vi "PvgeneratorOP400.vi"(8 "errin":errorcluster, 9 "BDD 3":T1, 10 "network":path, 11 "path in":path) -> (0 "sortie d'erreur":errorcluster caption="errout", 1 "network out":path, 2 "tout bon":bool, 3 "Chaîne":string)   [LabVIEW 2020]
uses:
  VG/IS30%.vi
  VG/PN.vi
  SubVI/OP400ZP_OCVmin.vi
  SubVI/OP400ZP_OCVmax.vi
  <vilib>/Utility/config.llb/NI_LVConfig.lvlib
panel:
  out "BDD 2":T2
  out "BDD":T1
  out "nombre de remplacements":i32
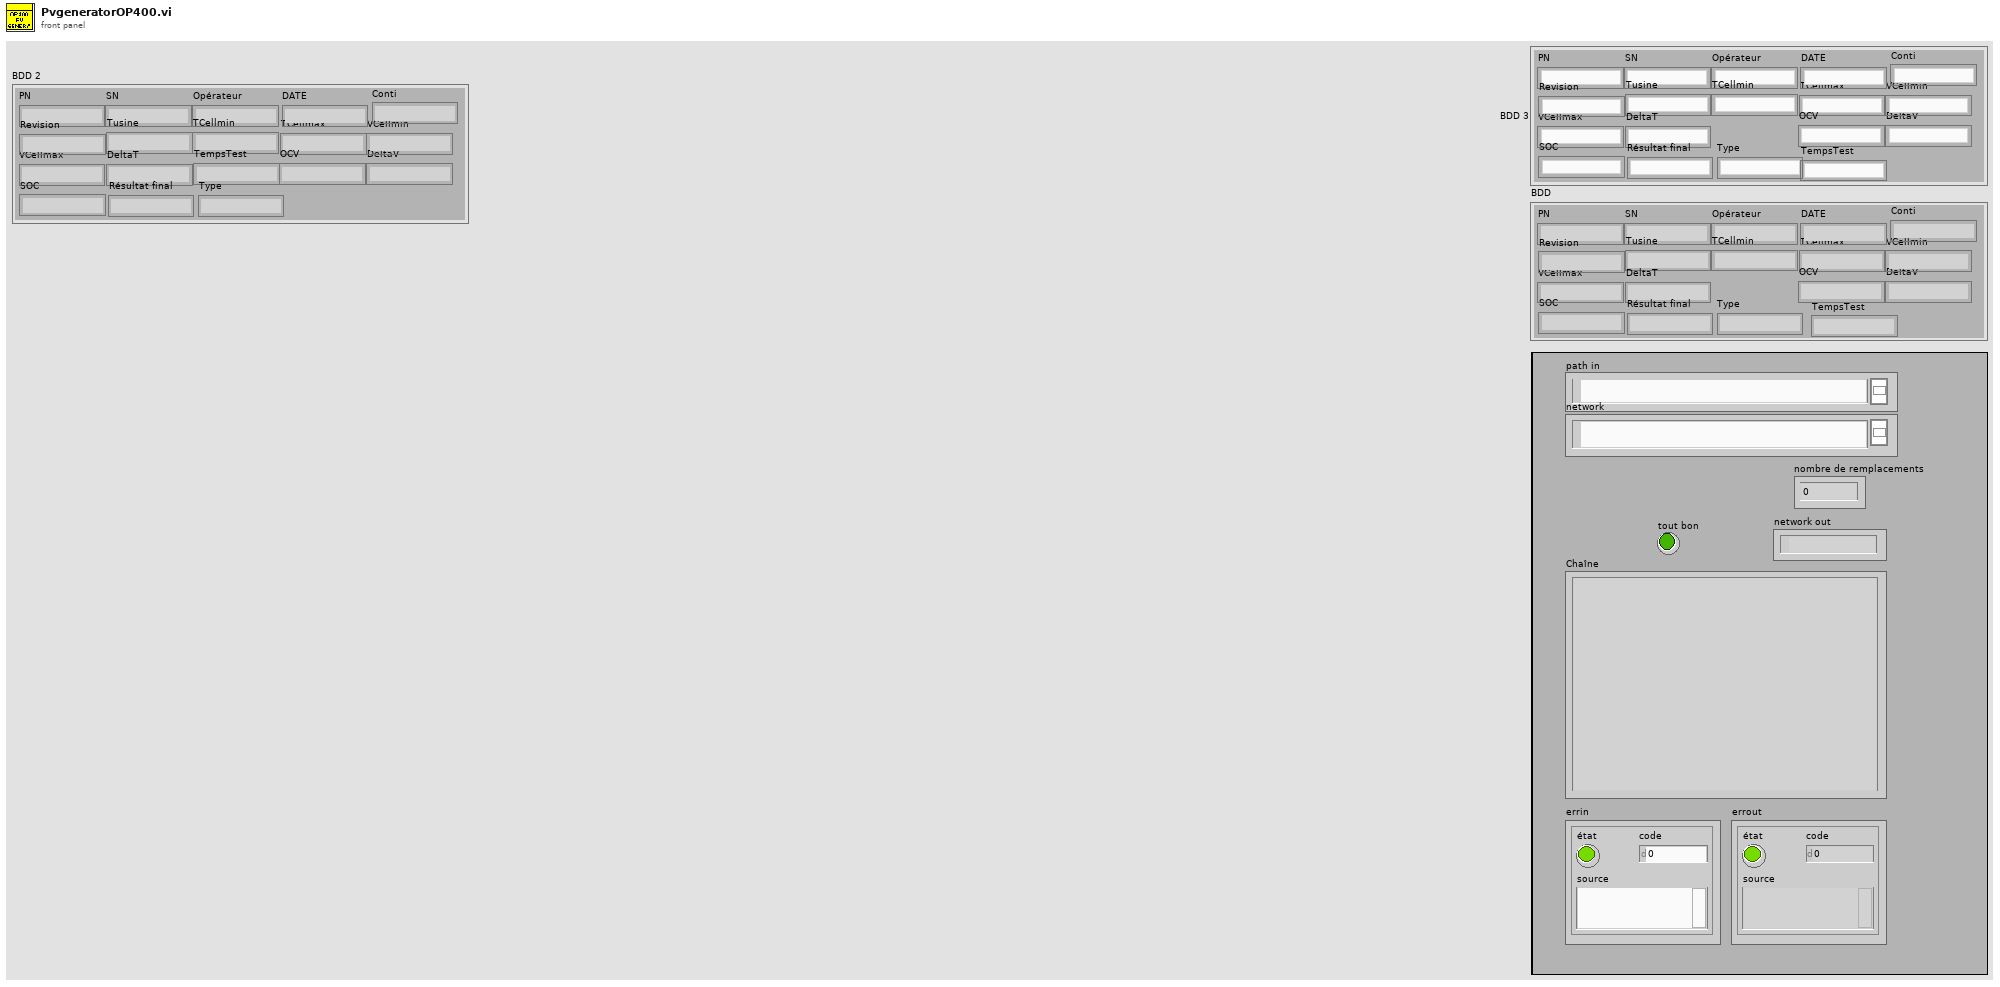
[diagram p1: front panel]
types:
  T1 = cluster{"PN":string, "SN":string, "Opérateur":string, "DATE":string, "Conti":string, "Revision":string, "Tusine":string, "TCellmin":string, "TCellmax":string, "VCellmin":string, "VCellmax":string, "DeltaT":string, "OCV":string, "DeltaV":string, "SOC":string, "Résultat final":string, "Type":string, "TempsTest":string}
  T2 = cluster{"PN":string, "SN":string, "Opérateur":string, "DATE":string, "Conti":string, "Revision":string, "Tusine":string, "TCellmin":string, "TCellmax":string, "VCellmin":string, "VCellmax":string, "DeltaT":string, "TempsTest":string, "OCV":string, "DeltaV":string, "SOC":string, "Résultat final":string, "Type":string}
  T3 = enum16{"open", "replace", "create", "open or create", "replace or create", "replace or create with confirmation"}
  T4 = typedef "NI_LVConfig.lvlib/Config Data RefNum.ctl" = refnum<k1>
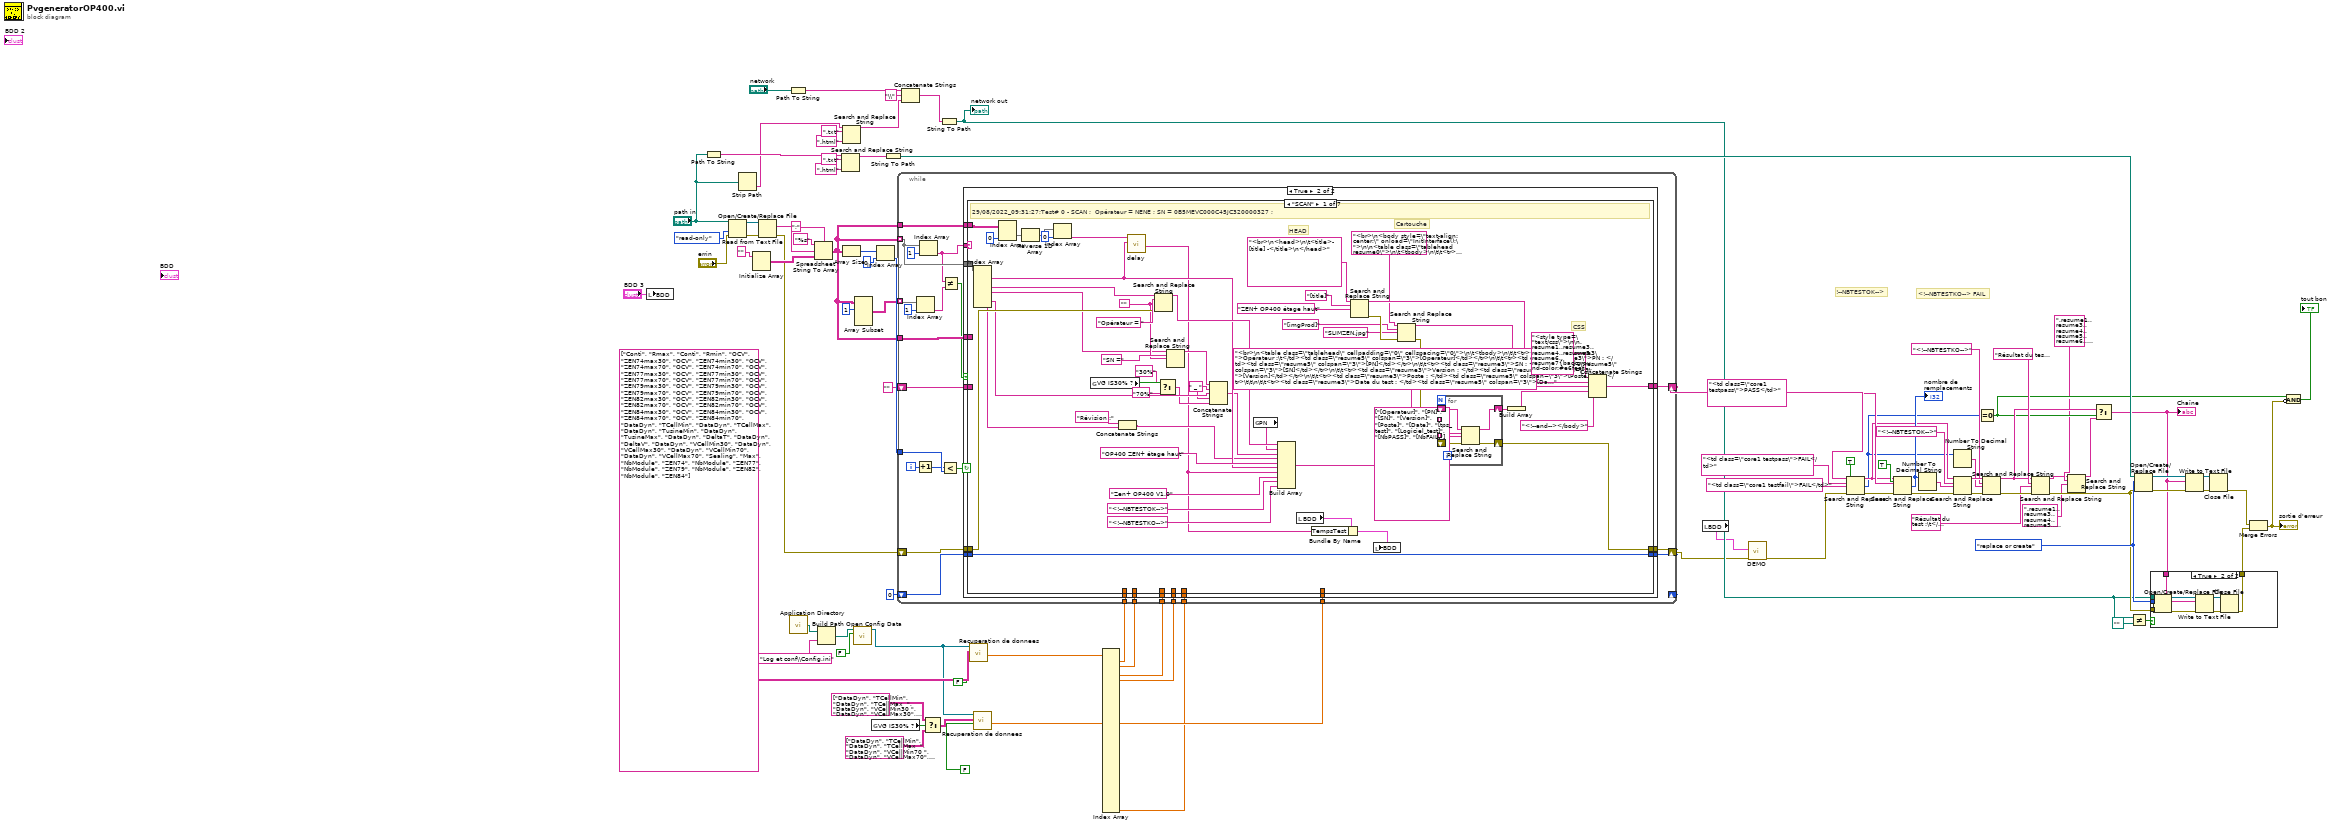
[diagram p0: block diagram]
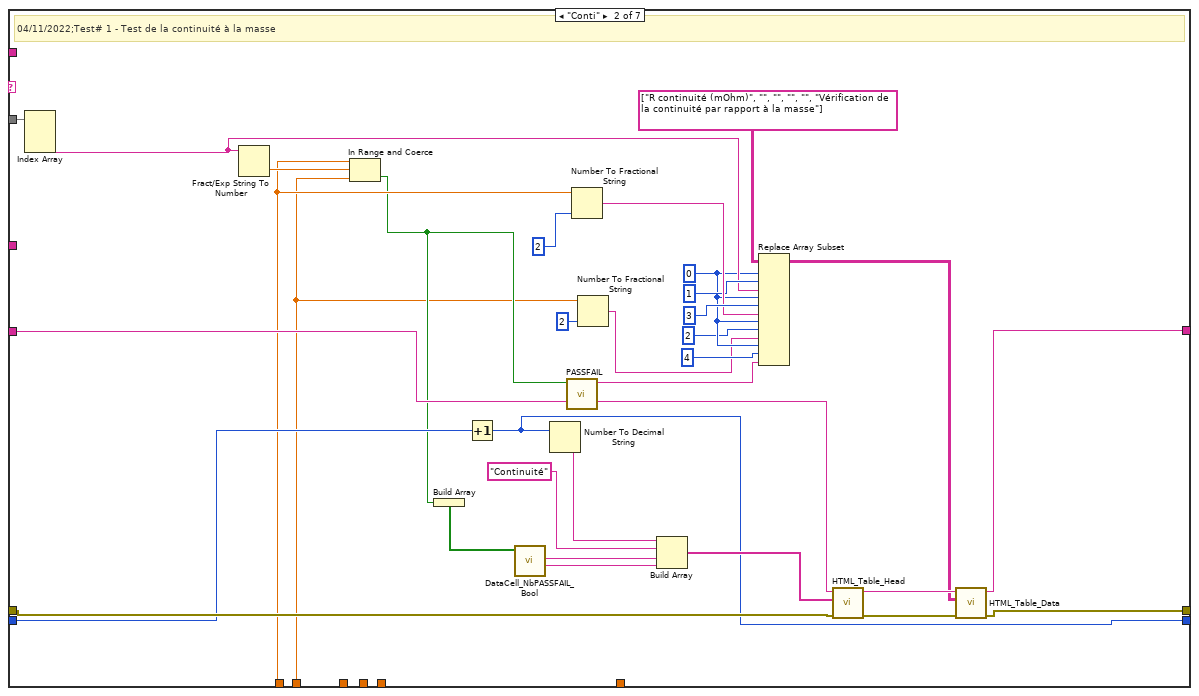
[diagram p3: hidden frame]
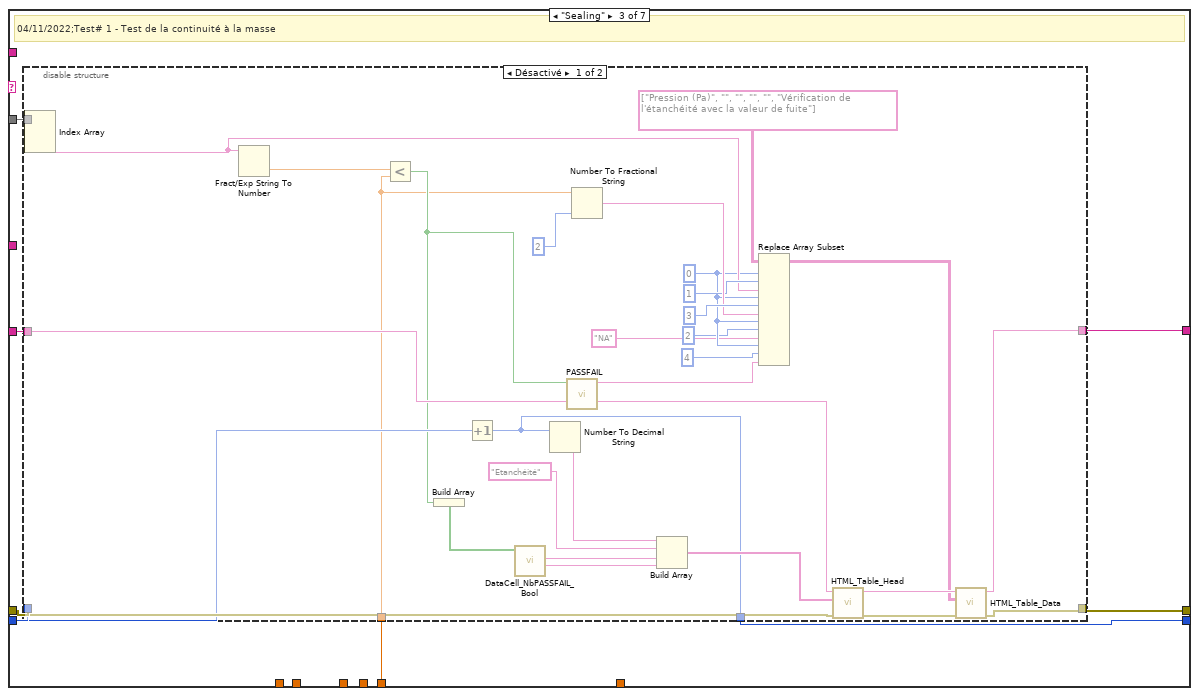
[diagram p4: hidden frame]
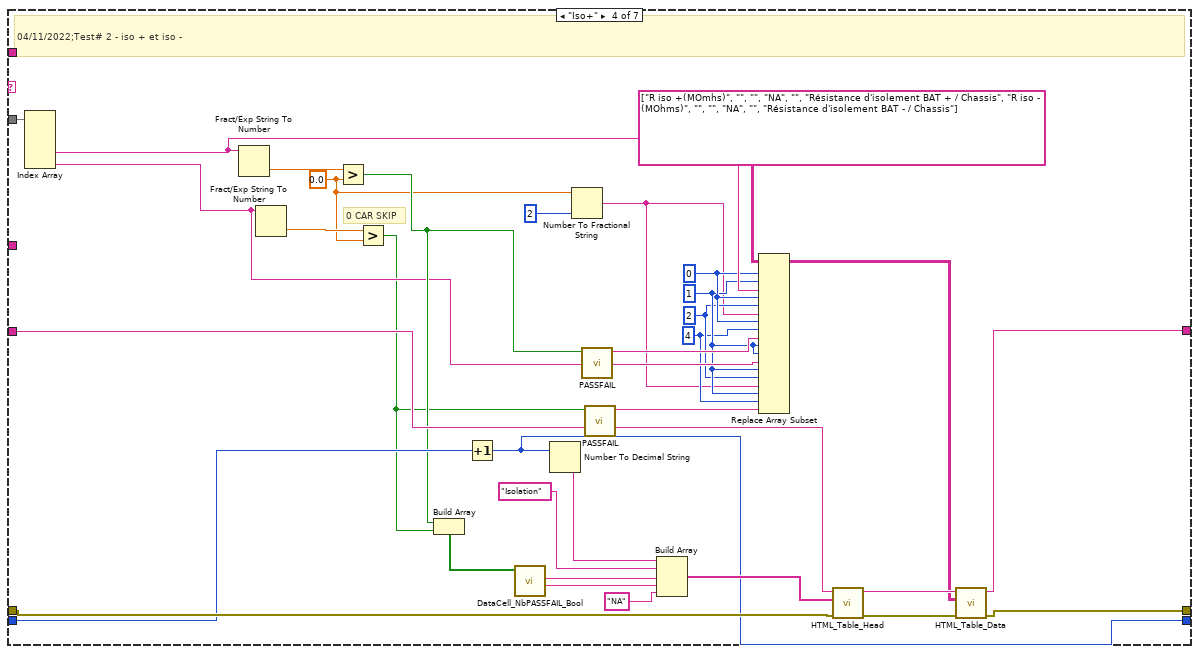
[diagram p6: hidden frame]
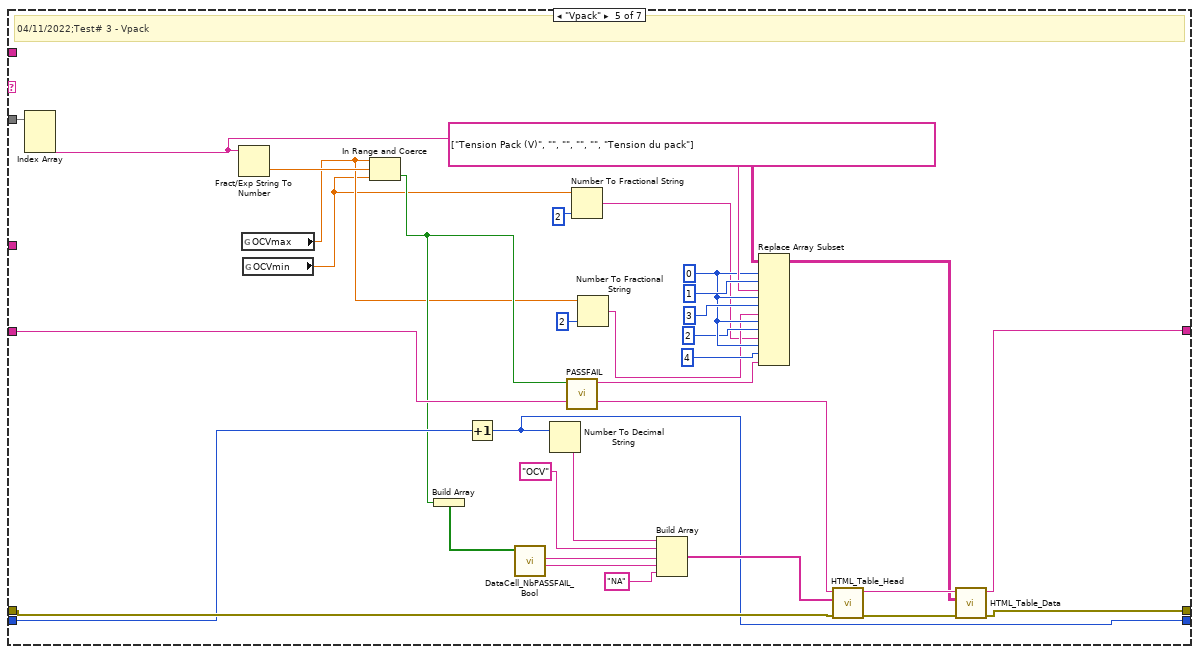
[diagram p7: hidden frame]
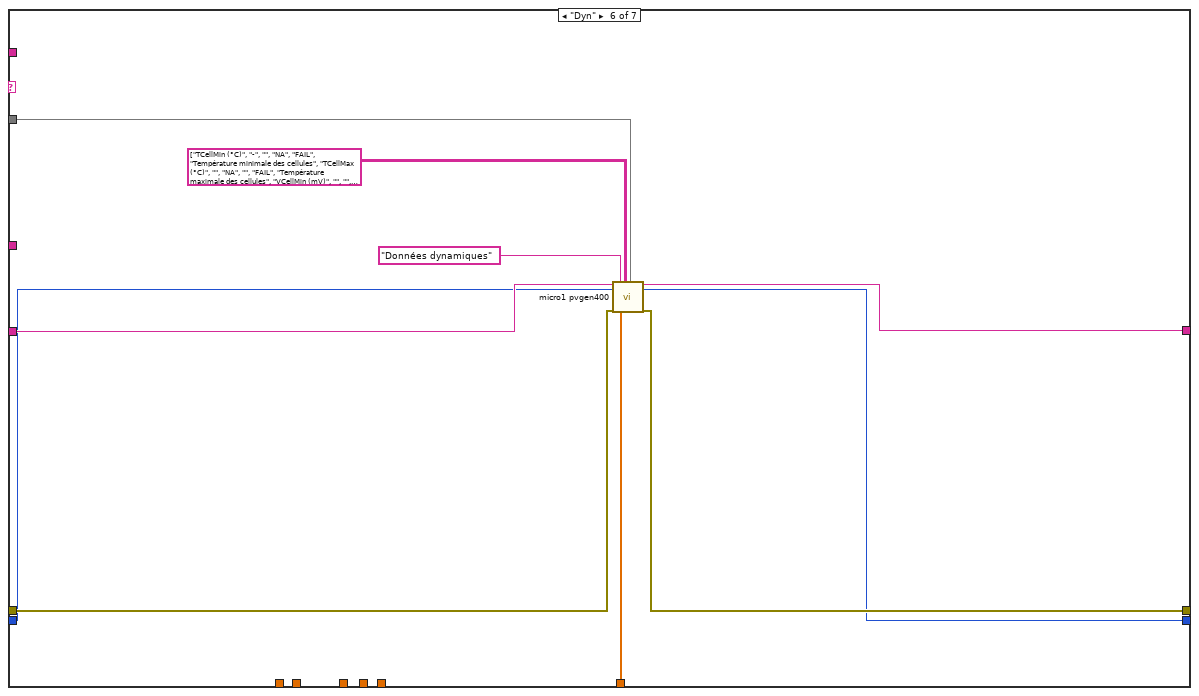
[diagram p8: hidden frame]
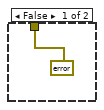
[diagram p10: hidden frame]
diagram:
  w56 = T3."replace or create" ("opération (0 : open)")
  # "<!--NBTESTKO--> FAIL"
  # "!--NBTESTOK-->"
  n1 = local write "BDD"("BDD 3") -> ()
  n2 = Path To String(path="path in") -> (string=w77:string)
  n3 = Open/Create/Replace File(file path (use dialog)="path in", error in="errin", access (0:read/write)=enum16{"read/write", "read-only", "write-only"}."read-only" ("accès (0 : read/write)")) -> (refnum out=w78:refnum<file>, error out=w94:errorcluster)  [unwired: 3 in, 1 out]
  n4 = Strip Path(path="path in") -> (name=w38:string)  [unwired: 1 out]
  n5 = Initialize Array("") -> (w92:string[][])  [unwired: 2 in]
  n6 = Read from Text File(file (use dialog)=w78, error in=w94) -> (text=w90:string, error out=w3:errorcluster)  [unwired: 2 in, 2 out]
  n7 = Path To String(path="network") -> (string=w37:string)
  n8 = call <vilib>:"Application Directory.vi"() -> ("Application Directory"=w29:path)
  n9 = Spreadsheet String To Array(delimiter (Tab)=";" ("séparateur (Tabulation)"), format string="%s" ("chaîne de format"), spreadsheet string=w90, array type (2D Dbl)=w92) -> (array=w14:string[][])
  n10 = Build Path(base path=w29, name or relative path="Log et conf\\Config.ini") -> (appended path=w32:path)
  n11 = Search and Replace String(input string=w77, search string=".txt" ("chaîne recherchée"), replace string=".html" ("chaîne de remplacement (\"\")")) -> (result string=w74:string)  [unwired: 5 in, 3 out]
  n12 = Search and Replace String(input string=w38, search string=".txt" ("chaîne recherchée"), replace string=".html" ("chaîne de remplacement (\"\")")) -> (result string=w35:string)  [unwired: 5 in, 3 out]
  n13 = Array Size(array=w14) -> (size(s)=w88:i32[])
  n14 = call <vilib>:"Open Config Data.vi"("create file if necessary (T)"=FALSE, "configuration file path"=w32) -> ("refnum"=w20:T4)  [unwired: 7 in, 2 out]
  n15 = Array Subset(array=w14, index (row)=1 ("indice")) -> (w12:string[][])  [unwired: 3 in]
  n16 = global read "IS30%.vi" "VG IS30% ?"() -> (w11:bool)
  n17 = Index Array(array=w88, index=0 ("indice")) -> (element=w86:i32)
  n18 = String To Path(string=w74) -> (path=w73:path)
  n19 = Concatenate Strings(w37, "\\" ("chaîne"), w35) -> (w34:string)
  n20 = Select(t=string[][] [["DataDyn", "TCellMin"], ["DataDyn", "TCellMax  "], ["DataDyn", "VCellMin30 "], ["DataDyn", "VCellMax30"], ["DataDyn", "TusineMax"], ["DataDyn", "TusineMin"], ["DataDyn", "DeltaT "], ["DataDyn", "DeltaV "]], s=w11, f=string[][] [["DataDyn", "TCellMin"], ["DataDyn", "TCellMax  "], ["DataDyn", "VCellMin70 "], ["DataDyn", "VCellMax70"], ["DataDyn", "TusineMax"], ["DataDyn", "TusineMin"], ["DataDyn", "DeltaT "], ["DataDyn", "DeltaV "]]) -> (s? t:f=w8:string[][])
  n21 = String To Path(string=w34) -> (path=w6:path)
  "network out" <- w6
  n22 = call "Recuperation de donnees.vi"("Est-ce un string?"=FALSE, "Array in"=string[][] [["Conti", "Rmax"], ["Conti", "Rmin"], ["OCV", "ZEN74max30"], ["OCV", "ZEN74min30"], ["OCV", "ZEN74max70"], ["OCV", "ZEN74min70"], ["OCV", "ZEN77max30"], ["OCV", "ZEN77min30"], ["OCV", "ZEN77max70"], ["OCV", "ZEN77min70"], ["OCV", "ZEN79max30"], ["OCV", "ZEN79min30"], ["OCV", "ZEN79max70"], ["OCV", "ZEN79min70"], ["OCV", "ZEN82max30"], ["OCV", "ZEN82min30"], ["OCV", "ZEN82max70"], ["OCV", "ZEN82min70"], ["OCV", "ZEN84max30"], ["OCV", "ZEN84min30"], ["OCV", "ZEN84max70"], ["OCV", "ZEN84min70"], ["DataDyn", "TCellMin"], ["DataDyn", "TCellMax"], ["DataDyn", "TusineMin"], ["DataDyn", "TusineMax"], ["DataDyn", "DeltaT"], ["DataDyn", "DeltaV"], ["DataDyn", "VCellMin30"], ["DataDyn", "VCellMax30"], ["DataDyn", "VCellMin70"], ["DataDyn", "VCellMax70"], ["Sealing", "Max"], ["NbModule", "ZEN74"], ["NbModule", "ZEN77"], ["NbModule", "ZEN79"], ["NbModule", "ZEN82"], ["NbModule", "ZEN84"]], "Refnum in"=w20) -> ("Array"=w26:dbl[])  [unwired: 7 in, 1 out]
  n23 = call "Recuperation de donnees.vi"("Est-ce un string?"=FALSE, "Array in"=w8, "Refnum in"=w20) -> ("Array"=w19:dbl[])  [unwired: 7 in, 1 out]
  n24 = Index Array(array=w26) -> (element #1=w25:dbl, element #2=w24:dbl, element #4=w23:dbl, element #5=w22:dbl, element #33=w7:dbl)  [unwired: 33 in, 28 out]
  n25 = while {
    tunnel: w86 -> [w119]
    tunnel: w14 -> [w116] mode=indexing
    shift-right: [w115] -> w2
    shift-left: w3 -> [w114]
    shift-right: [w108] -> w72
    shift-left: "" -> [w113]
    shift-right: [w111] -> _
    shift-left: 0 -> [w112]
    tunnel: w14 -> [w110]
    tunnel: w25 -> [w107]
    tunnel: w24 -> [w106]
    tunnel: w14 -> [w105]
    tunnel: w23 -> [w104]
    tunnel: w22 -> [w103]
    tunnel: w19 -> [w102]
    tunnel: w12 -> [w100] mode=indexing
    tunnel: w7 -> [w96]
    i -> [w120]
    stop <- w118 continue-if-true
    n26 = Index Array(array=w100, index=1 ("indice")) -> (element=w99:string)
    n27 = Increment(x=w120) -> (x+1=w109:i32)
    n28 = Index Array(array=w116, index=1 ("indice")) -> (element=w98:string)
    n29 = Less?(x=w109, y=w119) -> (x < y?=w118:bool)
    n30 = Not Equal?(x=w98, y=w99) -> (x != y?=w97:bool)
    n31 = case shown="True" w97 {
      tunnel: w116 -> [_ w139]
      tunnel: [w122 w138] -> w115
      tunnel: w114 -> [w122 w137]
      tunnel: w113 -> [w123 w136]
      tunnel: w112 -> [w121 w135]
      tunnel: [w121 w134] -> w111
      tunnel: w110 -> [_ w133]
      tunnel: [w123 w132] -> w108
      tunnel: w98 -> [_ w131]
      tunnel: w107 -> [_ w130]
      tunnel: w106 -> [_ w129]
      tunnel: w105 -> [_ w128]
      tunnel: w104 -> [_ w127]
      tunnel: w103 -> [_ w126]
      tunnel: w102 -> [_ w125]
      tunnel: w96 -> [_ w124]
      frame False {
      }
      frame True {
        n32 = case shown="\"SCAN\"" w131 {
          tunnel: w137 -> [w192 w224 w238 w294 w327 w344 w348]
          tunnel: w139 -> [w158 w225 w239 w295 w328 w340 _]
          tunnel: [w171 w223 w237 w293 w326 w343 w348] -> w138
          tunnel: w136 -> [_ w222 w236 w292 w325 w338 w346]
          tunnel: w135 -> [w170 w221 w235 w291 w324 w337 w347]
          tunnel: [w170 w220 w234 w290 w323 w336 w347] -> w134
          tunnel: w133 -> [_ _ _ _ _ _ _]
          tunnel: [w169 w219 w233 w289 w322 w342 w346] -> w132
          tunnel: w130 -> [_ w208 _ _ _ _ _]
          tunnel: w129 -> [_ w201 _ _ _ _ _]
          tunnel: w128 -> [w148 _ _ _ _ _ _]
          tunnel: w127 -> [_ _ _ _ _ _ _]
          tunnel: w126 -> [_ _ _ _ _ _ _]
          tunnel: w125 -> [_ _ _ _ _ w345 _]
          tunnel: w124 -> [_ _ w232 _ _ _ _]
          frame "SCAN" {
            w157 = " _ " ("chaîne")
            w165 = ""
            # "Cartouche"
            # "HEAD"
            # "CSS"
            # "29/08/2022_09:31:27;Test# 0 - SCAN ;  Opérateur = NENE ; SN = 0B5MEVC000C45JC320000327 ;"
            n33 = Index Array(array=w158) -> (element #1=w163:string, element #3=w168:string, element #4=w164:string, element #6=w159:string, element #7=w150:string)  [unwired: 7 in, 2 out]
            n34 = Index Array(array=w148, index (col)=0 ("disabled index (col)")) -> (element=w146:string[])  [unwired: 1 in]
            n35 = Reverse 1D Array(array=w146) -> (reversed array=w145:string[])
            n36 = Index Array(array=w145, index=0) -> (element=w143:string)
            n37 = global read "IS30%.vi" "VG IS30% ?"() -> (w156:bool)
            n38 = Concatenate Strings("Révision :", w150) -> (w149:string)
            n39 = call "delay.vi"("String"=w163, "String 2"=w143) -> ("Delay calculé"=w140:string)  [unwired: 9 in]
            n40 = Search and Replace String(input string=w168, search string="Opérateur = " ("chaîne recherchée"), replace string=w165, error in=w192) -> (result string=w167:string)  [unwired: 4 in, 3 out]
            n41 = Select(t="30%" ("chaîne recherchée"), s=w156, f="70%" ("cas faux")) -> (s? t:f=w155:string)
            n42 = Search and Replace String(input string=w164, search string="SN =" ("chaîne recherchée"), replace string=w165) -> (result string=w160:string)  [unwired: 5 in, 3 out]
            n43 = Concatenate Strings(w160, w157, w159, w157, w155) -> (w161:string)
            n44 = global read "PN.vi" "PN"() -> (w152:string)
            n45 = Build Array(w167, w152, w161, w149, "OP400 ZEN+ étage haut" ("chaîne"), w163, w140, "Zen+ OP400 V1.0" ("chaîne"), "<!--NBTESTOK-->" ("chaîne"), "<!--NBTESTKO-->" ("chaîne")) -> (w172:string[])
            n46 = local read "BDD"() -> (w142:T1)
            n47 = Bundle By Name(cluster=w142, "TempsTest"=w140) -> (w141:T1)
            n48 = Search and Replace String(input string="<br>\n<head>\n\t<title>- [title] -</title>\n</head>", search string="[title]" ("chaîne recherchée"), replace string="ZEN+ OP400 étage haut" ("Title")) -> (result string=w188:string, error out=w187:errorcluster)  [unwired: 5 in, 2 out]
            n49 = local write "BDD"(w141) -> ()
            n50 = Search and Replace String(input string="<br>\n<body style=\"text-align: center;\" onload=\"InitInterface();\">\n\n<table class=\"tablehead resume0\">\n\t<tbody>\n\t\t<tr>\n\t\t\t<td> <img src=\"[imgProd]\" style=\"width:194px;height:100px\" class=\"left\"></td>\n\t\t\t<td> <div class=\"center\">PROCES VERBAL DE TEST AUTOMATIQUE</div><div class=\"center\">Zen+ OP400</div><br class=\"center\"><div class=\"center\">Forseepower</div></td>\n\t\t\t<td> <img src=\"LOGO FORSEE.png\" style=\"width:194px;height:100px\"  class=\"right\"></td>\n\t\t</tr>\n\t</tbody>\n</table>", search string="[imgProd]", replace string="SLIMZEN.jpg" ("imgProd"), error in=w187) -> (result string=w185:string, error out=w182:errorcluster)  [unwired: 4 in, 2 out]
            n51 = for {
              shift-right: [w198] -> w181
              shift-left: "<br>\n<table class=\"tablehead\" cellpadding=\"0\" cellspacing=\"0\">\n\t<tbody>\n\t\t<tr><td class=\"resume3\">Opérateur :\t</td><td class=\"resume5\" colspan=\"3\">[Operateur]</td></tr>\n\t\t<tr><td class=\"resume3\">PN : </td><td class=\"resume5\" colspan=\"3\">[PN]</td></tr>\n\t\t<tr><td class=\"resume3\">SN : </td><td class=\"resume5\" colspan=\"3\">[SN]</td></tr>\n\t\t<tr><td class=\"resume3\">Version : </td><td class=\"resume5\" colspan=\"3\">[Version]</td></tr>\n\t\t<tr><td class=\"resume3\">Poste : </td><td class=\"resume5\" colspan=\"3\">[Poste]</td></tr>\t\t\n\t\t<tr><td class=\"resume3\">Date du test : </td><td class=\"resume5\" colspan=\"3\">[Date]</td></tr>\n\t\t<tr><td class=\"resume3\">Temps de test : </td><td class=\"resume5\" colspan=\"3\">[tps_test]</td></tr>\n\t\t<tr><td class=\"resume3\">Logiciel de test :\t</td><td class=\"resume5\" colspan=\"3\">[Logiciel_test]</td></tr>\n\t\t<tr><td class=\"resume3\">Résultat du test :\t</td><td class=\"resume5\" colspan=\"3\"><div><span style=\"float:left\" id=\"result\"><font size = \"5pt\" color=\"green\"><b>CONFORME</b></font><b><font size = \"5pt\"> ( </font><font size = \"5pt\" color=\"green\">[NbPASS] PASS </font>  <font size = \"5pt\"> / </font><font size = \"5pt\" color=\"red\">[NbFAIL] FAIL</font> <font size = \"5pt\"> ) </font></b></span></div></td></tr>\n\t</tbody>\n</table>" -> [w199]
              tunnel: string[] ["[Operateur]", "[PN]", "[SN]", "[Version]", "[Poste]", "[Date]", "[tps_test]", "[Logiciel_test]", "[NbPASS]", "[NbFAIL]"] -> [w195] mode=indexing
              tunnel: w172 -> [w194] mode=indexing
              shift-right: [w196] -> w171
              shift-left: w182 -> [w197]
              n52 = Search and Replace String(input string=w199, search string=w195, replace string=w194, error in=w197) -> (result string=w198:string, error out=w196:errorcluster)  [unwired: 4 in, 2 out]
            }
            n53 = Build Array(w181) -> (w180:string[])
            n54 = Concatenate Strings("<style type=\"text/css\">\n\n.resume1,.resume3,.resume4,.resume5,.resume6,.resume7{background-color:#e6feef;padding:7px;border:1px solid black;}\n.resume0{border:1px solid black;background-color:#e6feef;font-weight: bold;padding:0px;text-align: center;}\n.resume1{width:350px;text-align:right;font-weight:bold;}\n.resume3{width:350px;text-align:right;border-top:0px solid black;font-weight:bold;}\n.resume4{border-left:0px solid black;width:290px;}\n.resume5{width:290px;border-left:0px solid black;border-top:0px solid black;}\n.resume6{border-left:0px solid black;width:60px;}\n.resume7{border-left:0px solid black;border-top:0px solid black;width:60px;}\n.title1{text-align: left;background-color:#e6f4fe;padding:10px;border:1px solid #101010;}\n.title2{width: 30px;text-align: center;background-color:#e6f4fe;padding:1px;border:1px solid #101010;border-left:0px solid black;font-weight: bold;}\n.title2 a:link{text-decoration:none;}\n.entete0,.entete1,.entete2,.time2{text-align: center;background-color:#feeec9;padding:7px;border:1px solid black;font-weight: bold;}\n.entete0{width:45px;border-right:0px solid black;}\n.entete1{width:505px;}\n.entete2{width:95px;border-right:0px solid black;}\n.time2{border-left:0px solid black;width:145px;font-size:11px;}\n.core0,.core1,.core2,.core3,.core4,.time{text-align: center;background-color:#fafed3;padding:7px;border:1px solid black;}\n.core0, .core1,.core3,.core4{width:95px;border-top:0px solid black;border-right:0px solid black;}\n.core0{width:45px;}\n.core2{border-top:0px solid black;width:505px;}\n.core3{width:200px;}\n.core4{width:300px;}\n.time{width:145px;border-top:0px solid black;border-left:0px solid black;font-size:11px;}\n.false .core0,.false .core1,.false .core2,.false .core3,.false .core4,.false .time{background-color:#f4f4f4;}\n.false .entete0,.false .entete1,.false .entete2,.false .time2{background-color:#dadada;}\n.false .title1,.false .title2,.false .resultentete .testpass,.false .resultentete .testfail,.false .resultentete .testtime{background-color:#c5cac9;color: blue;}\n.false .title2 a:link{text-decoration:none;color: blue;}\n.comment1,.comment2,.time3{width: 890px;background-color:#e9e8e9;padding:7px;border:1px solid black;border-top:0px solid black;text-align:left;}\n.comment2{border-right:0px solid black;width: 45px;text-align: center;}\n.time3{width: 145px;border-left:0px solid black;font-size:11px;}\n.fixe1{background: -moz-linear-gradient(center top , #101010 10%, #555555 80%) repeat scroll 0 0 transparent;background: -webkit-gradient(linear, left top, left bottom, from(#101010), to(#555555));border:2px solid orange;position : fixed;margin-top:20px;display:none;overflow-y:scroll;max-height:350px;text-shadow: 0px 0px 0 #333333;text-align:left;font-size:10px;padding:10px;margin-left:-162px;border-radius: 15px 15px 15px 15px;}\n.menufixe, .menufixelock{background: -moz-linear-gradient(center top , #101010 80%, transparent 20%) repeat scroll 0 0 transparent;background: -webkit-gradient(linear, left top, left bottom, from(#101010), color-stop(0.65, #101010), to(transparent)) repeat scroll 0 0 transparent;margin: -52px 0px 0px -9px;width:100%;position:fixed;height:55px;-moz-transition: margin 1s;-webkit-transition: margin 1s;}\n.menufixelock, .menufixe:hover{margin: -9px 0px 0px -9px;}\n.lockmenu, .separation,.separationmenu{text-align:center;background: -moz-linear-gradient(center top , #555555 10%, #111111 80%) repeat scroll 0 0 transparent;background: -webkit-gradient(linear, left top, left bottom, from(#555555), to(#111111));border: 1px solid white;border-radius: 10px 10px 10px 10px;box-shadow: 0 -1px 1px #555555 inset;color: #999999;font-weight: bold;width: 100px;padding: 2px;text-decoration: none;}\n.tablehead{width: 1000px;font-family: Verdana;font-size: 12px;margin-left: auto;margin-right: auto;}\n.tablenull{font-family: Verdana;font-size: 11px;margin-left: auto;margin-right: auto;}\n.separationmenu:hover div{display: inline;}\n.lockmenu:hover, .separation:hover,.separationmenu:hover{border: 1px solid orange;cursor:pointer;}\n.lockmenu:hover{border: 1px solid red;cursor:pointer;}\n.separationright{padding:10px;}\ndiv a:link{text-decoration:none;color:#cbcbcb;}\ndiv a:hover{text-decoration:underline;color:#cbcbcb;}\nspan a:link{text-decoration:none;color:#cbcbcb;}\nspan a:hover{text-decoration:none;color:#cbcbcb;}\n.false{color: blue;}\n.testpass{color: green;font-weight: bold;}\n.testfail{color: red;font-weight: bold;}\n.testtime{color: blue;font-weight: bold;}\n.resultentete{font-weight: bold;font-size: 11px;min-width: 200px;text-align:right;}\n.infohard{border: 1px solid black;background-color: white;text-align: center;width: 16px;height: 16px;border-radius: 5px;font-weight: bold;box-shadow: 0 -1px 2px #555555 inset;}\n.infohard:hover{background-color:#feeec9;cursor:pointer;}\n.footerhard{padding-top:30px;}\n.confighard{font-size:10px;width:110px;}\n.circlemain{margin-left:auto;margin-right:auto;}\n.circletext,.circleform{padding-top: 3px;text-align:center;font-size: 10px;width:200px;}\n.circleform{padding-bottom: 3px;padding-top: 1px;}\n.circle{border: 1px solid black;border-collapse: collapse;border-radius: 15px;box-shadow: 1px 1px 0 #505050;height: 15px;width: 15px;display:inline-block;}\n.bookmarkon, .bookmarkoff{background-color: yellow;border: 1px solid black;border-collapse: collapse;border-radius: 10px 10px 10px 10px;box-shadow: 1px 1px 0 #505050;height: 12px;width: 12px;position: absolute;margin-left:22px;cursor: help;}\n.bookmarkoff{background-color: transparent;border: 1px solid #CECECE;box-shadow: none;cursor: copy;}\n.false .bookmarkoff{background-color: transparent;border: 1px solid #E6E1E1;box-shadow: none;cursor: copy;}\n.bookmarkmaster{height: 15px;margin-right: 12px;width: 60px;}\n.bookmarkmaster:hover .bookmarkprev,.bookmarkmaster:hover .bookmarksuiv{display:block;}\n.bookmarkprev, .bookmarksuiv {cursor: pointer;font-size: 25px;font-weight: bold;margin-top: -10px;position: absolute;display:none;}\n.bookmarkprev{margin-left: 2px;}\n.bookmarksuiv{margin-left: 43px;}\n.plus, .moins{background-color: #F4F4F4;border: 1px solid #848484;border-radius: 20px;color: #848484;font-family: arial;font-size: 16px;font-weight: bold;height: 20px;margin-left: 4px;text-align: center;width: 20px;}\n.moins{font-size: 15px;}\n.plus:hover, .moins:hover{background-color: #DADADA;border: 1px solid black;color: black;cursor:pointer;}\n.backtothetop {position: fixed; right: 50%; margin-right: -555px; bottom: 10px; font-size: 35px; font-weight: bold; border: 1px solid #7D7B91; width: 40px; height: 40px; line-height:52px; text-align: center;border-radius: 8px; opacity: 0.25; background-color: #F5F5F5; color:#7D7B91;}\n.backtothetop:hover {opacity: 1; cursor:pointer;}\n.libversion {font-size: 8px;font-weight: normal;padding-right: 10px;text-align: right;}\n.lockmenu {width: 18px;font-size: 12px;}\n.left {display: block; margin-left: 1px;margin-right: auto;}\n.right {display: block; margin-right: 1px;margin-left: auto;}\n.center {display: block; margin-left: auto;margin-right: auto;}\n\n</style>", w188, w185, w180, "<!--end--></body>") -> (w169:string)
          }
          frame "Conti" {
            w205 = 0 ("index (row)")
            # "04/11/2022;Test# 1 - Test de la continuité à la masse"
            n55 = Index Array(array=w225) -> (element #3=w210:string)  [unwired: 3 in, 2 out]
            n56 = Fract/Exp String To Number(string=w210) -> (number=w209:dbl)  [unwired: 3 in, 1 out]
            n57 = In Range and Coerce(upper limit=w208, x=w209, lower limit=w201) -> (In Range?=w203:bool)  [unwired: 1 out]
            n58 = Build Array(w203) -> (w217:bool[])
            n59 = Increment(x=w221) -> (x+1=w220:i32)
            n60 = call "DataCell_NbPASSFAIL_Bool.vi"("Tableau en entrée"=w217) -> ("Chaîne"=w215:string, "Chaîne 2"=w216:string)  [unwired: 8 in, 1 out]
            n61 = Number To Decimal String(number=w220) -> (decimal integer string=w227:string)  [unwired: 1 in]
            n62 = call "PASSFAIL.vi"("E"=w203) -> ("S"=w207:string)  [unwired: 10 in]
            n63 = Number To Fractional String(number=w208, precision (6)=i16 2) -> (F-format string=w213:string)  [unwired: 2 in]
            n64 = Number To Fractional String(number=w201, precision (6)=i16 2) -> (F-format string=w200:string)  [unwired: 2 in]
            n65 = Build Array(w227, "Continuité" ("élément"), w216, w215) -> (w230:string[])
            n66 = Replace Array Subset(array=string[][] [["R continuité (mOhm)", "", "", "", "", "Vérification de la continuité par rapport à la masse"]] ("Tableau"), new element #1=w210, index (row) #1=w205, index (col) #1=1 ("disabled index (col)"), new element #2=w213, index (row) #2=w205, index (col) #2=3 ("disabled index (col)"), new element #3=w200, index (row) #3=w205, index (col) #3=2 ("disabled index (col)"), new element #4=w207, index (row) #4=w205, index (col) #4=4 ("disabled index (col)")) -> (w218:string[][])
            n67 = call "HTML_Table_Head.vi"("entrée d'erreur (pas d'erreur)"=w224, "Tableau"=w230, "chaîne en entrée"=w222) -> ("sortie d'erreur"=w229:errorcluster, "result string"=w228:string)  [unwired: 7 in]
            n68 = call "HTML_Table_Data.vi"("entrée d'erreur (pas d'erreur)"=w229, "Tableau"=w218, "chaîne en entrée"=w228) -> ("sortie d'erreur"=w223:errorcluster, "result string"=w219:string)  [unwired: 7 in]
          }
          frame "Sealing" {
            # "04/11/2022;Test# 1 - Test de la continuité à la masse"
            n69 = disable-structure shown="Désactivé" {
              disable-tunnel: w239 -> [w263 _]
              disable-tunnel: w238 -> [w262 _]
              disable-tunnel: [w261 _] -> w237
              disable-tunnel: w236 -> [w260 _]
              disable-tunnel: w235 -> [w259 _]
              disable-tunnel: [w258 _] -> w234
              disable-tunnel: [w257 _] -> w233
              disable-tunnel: w232 -> [w240 _]
              frame Disabled {
                w244 = 0 ("index (row)")
                n70 = Index Array(array=w263) -> (element #3=w248:string)  [unwired: 3 in, 2 out]
                n71 = Fract/Exp String To Number(string=w248) -> (number=w247:dbl)  [unwired: 3 in, 1 out]
                n72 = Less?(x=w247, y=w240) -> (x < y?=w242:bool)
                n73 = Build Array(w242) -> (w255:bool[])
                n74 = Increment(x=w259) -> (x+1=w258:i32)
                n75 = call "DataCell_NbPASSFAIL_Bool.vi"("Tableau en entrée"=w255) -> ("Chaîne"=w253:string, "Chaîne 2"=w254:string)  [unwired: 8 in, 1 out]
                n76 = Number To Decimal String(number=w258) -> (decimal integer string=w265:string)  [unwired: 1 in]
                n77 = call "PASSFAIL.vi"("E"=w242) -> ("S"=w246:string)  [unwired: 10 in]
                n78 = Number To Fractional String(number=w240, precision (6)=i16 2) -> (F-format string=w251:string)  [unwired: 2 in]
                n79 = Build Array(w265, "Etanchéité" ("élément"), w254, w253) -> (w268:string[])
                n80 = Replace Array Subset(array=string[][] [["Pression (Pa)", "", "", "", "", "Vérification de l'étanchéité avec la valeur de fuite"]] ("Tableau"), new element #1=w248, index (row) #1=w244, index (col) #1=1 ("disabled index (col)"), new element #2=w251, index (row) #2=w244, index (col) #2=3 ("disabled index (col)"), new element #3="NA" ("nouvel élément/sous-tableau"), index (row) #3=w244, index (col) #3=2 ("disabled index (col)"), new element #4=w246, index (row) #4=w244, index (col) #4=4 ("disabled index (col)")) -> (w256:string[][])
                n81 = call "HTML_Table_Head.vi"("entrée d'erreur (pas d'erreur)"=w262, "Tableau"=w268, "chaîne en entrée"=w260) -> ("sortie d'erreur"=w267:errorcluster, "result string"=w266:string)  [unwired: 7 in]
                n82 = call "HTML_Table_Data.vi"("entrée d'erreur (pas d'erreur)"=w267, "Tableau"=w256, "chaîne en entrée"=w266) -> ("sortie d'erreur"=w261:errorcluster, "result string"=w257:string)  [unwired: 7 in]
              }
              frame Enabled {
              }
            }
          }
          frame "Iso+" {
            w270 = 0.0 ("y")
            w274 = 4 ("disabled index (col)")
            w275 = 2 ("disabled index (col)")
            w276 = 1 ("disabled index (col)")
            w282 = 0 ("index (row)")
            # "0 CAR SKIP"
            # "04/11/2022;Test# 2 - iso + et iso -"
            n83 = Index Array(array=w295) -> (element #3=w283:string, element #5=w277:string)  [unwired: 5 in, 3 out]
            n84 = Fract/Exp String To Number(string=w283) -> (number=w281:dbl)  [unwired: 3 in, 1 out]
            n85 = Fract/Exp String To Number(string=w277) -> (number=w279:dbl)  [unwired: 3 in, 1 out]
            n86 = Greater?(x=w281, y=w270) -> (0:w280:bool)
            n87 = Greater?(x=w279, y=w270) -> (0:w272:bool)
            n88 = Build Array(w280, w272) -> (w287:bool[])
            n89 = Increment(x=w291) -> (x+1=w290:i32)
            n90 = call "DataCell_NbPASSFAIL_Bool.vi"("Tableau en entrée"=w287) -> ("Chaîne"=w285:string, "Chaîne 2"=w286:string)  [unwired: 8 in, 1 out]
            n91 = Number To Decimal String(number=w290) -> (decimal integer string=w298:string)  [unwired: 1 in]
            n92 = Number To Fractional String(number=w270, precision (6)=i16 2) -> (F-format string=w273:string)  [unwired: 2 in]
            n93 = call "PASSFAIL.vi"("E"=w280) -> ("S"=w278:string)  [unwired: 10 in]
            n94 = call "PASSFAIL.vi"("E"=w272) -> ("S"=w271:string)  [unwired: 10 in]
            n95 = Build Array(w298, "Isolation" ("élément"), w286, w285, "NA" ("élément")) -> (w301:string[])
            n96 = Replace Array Subset(array=string[][] [["R iso +(MOmhs)", "", "", "NA", "", "Résistance d'isolement BAT + / Chassis"], ["R iso - (MOhms)", "", "", "NA", "", "Résistance d'isolement BAT - / Chassis"]] ("Tableau"), new element #1=w283, index (row) #1=w282, index (col) #1=w276, new element #2=w273, index (row) #2=w282, index (col) #2=w275, new element #3=w278, index (row) #3=w282, index (col) #3=w274, new element #4=w277, index (row) #4=w276, index (col) #4=w276, new element #5=w273, index (row) #5=w276, index (col) #5=w275, new element #6=w271, index (row) #6=w276, index (col) #6=w274) -> (w288:string[][])
            n97 = call "HTML_Table_Head.vi"("entrée d'erreur (pas d'erreur)"=w294, "Tableau"=w301, "chaîne en entrée"=w292) -> ("sortie d'erreur"=w300:errorcluster, "result string"=w299:string)  [unwired: 7 in]
            n98 = call "HTML_Table_Data.vi"("entrée d'erreur (pas d'erreur)"=w300, "Tableau"=w288, "chaîne en entrée"=w299) -> ("sortie d'erreur"=w293:errorcluster, "result string"=w289:string)  [unwired: 7 in]
          }
          frame "Vpack" {
            w310 = 0 ("index (row)")
            # "04/11/2022;Test# 3 - Vpack"
            n99 = Index Array(array=w328) -> (element #3=w314:string)  [unwired: 3 in, 2 out]
            n100 = Fract/Exp String To Number(string=w314) -> (number=w313:dbl)  [unwired: 3 in, 1 out]
            n101 = global read "OP400ZP_OCVmax.vi" "OCVmax"() -> (w304:dbl)
            n102 = global read "OP400ZP_OCVmin.vi" "OCVmin"() -> (w303:dbl)
            n103 = In Range and Coerce(upper limit=w304, x=w313, lower limit=w303) -> (In Range?=w308:bool)  [unwired: 1 out]
            n104 = Build Array(w308) -> (w320:bool[])
            n105 = Increment(x=w324) -> (x+1=w323:i32)
            n106 = call "DataCell_NbPASSFAIL_Bool.vi"("Tableau en entrée"=w320) -> ("Chaîne"=w318:string, "Chaîne 2"=w319:string)  [unwired: 8 in, 1 out]
            n107 = Number To Decimal String(number=w323) -> (decimal integer string=w331:string)  [unwired: 1 in]
            n108 = call "PASSFAIL.vi"("E"=w308) -> ("S"=w312:string)  [unwired: 10 in]
            n109 = Number To Fractional String(number=w303, precision (6)=i16 2) -> (F-format string=w305:string)  [unwired: 2 in]
            n110 = Number To Fractional String(number=w304, precision (6)=i16 2) -> (F-format string=w306:string)  [unwired: 2 in]
            n111 = Build Array(w331, "OCV" ("élément"), w319, w318, "NA" ("élément")) -> (w334:string[])
            n112 = Replace Array Subset(array=string[][] [["Tension Pack (V)", "", "", "", "", "Tension du pack"]] ("Tableau"), new element #1=w314, index (row) #1=w310, index (col) #1=1 ("disabled index (col)"), new element #2=w306, index (row) #2=w310, index (col) #2=3 ("disabled index (col)"), new element #3=w305, index (row) #3=w310, index (col) #3=2 ("disabled index (col)"), new element #4=w312, index (row) #4=w310, index (col) #4=4 ("disabled index (col)")) -> (w321:string[][])
            n113 = call "HTML_Table_Head.vi"("entrée d'erreur (pas d'erreur)"=w327, "Tableau"=w334, "chaîne en entrée"=w325) -> ("sortie d'erreur"=w333:errorcluster, "result string"=w332:string)  [unwired: 7 in]
            n114 = call "HTML_Table_Data.vi"("entrée d'erreur (pas d'erreur)"=w333, "Tableau"=w321, "chaîne en entrée"=w332) -> ("sortie d'erreur"=w326:errorcluster, "result string"=w322:string)  [unwired: 7 in]
          }
          frame "Dyn" {
            n115 = call "micro1 pvgen400.vi"("FluxStrIn"=w338, "Numin"=w337, "errin"=w344, "testlabel"="Données dynamiques", "Data limit"=w345, "tab ref"=string[][] [["TCellMin (°C)", "-", "", "NA", "FAIL", "Température minimale des cellules"], ["TCellMax (°C)", "", "NA", "", "FAIL", "Température maximale des cellules"], ["VCellMin (mV)", "", "", "NA", "FAIL", "Tension minimale des cellues"], ["VCellMax (mV)", "", "NA", "", "FAIL", "Tension maximale des cellues"], ["Tusine (°C)", "", "", "", "FAIL", "Température de l'usine"], ["DeltaT (°C)", "", "NA", "", "FAIL", "Différence maximale de température entre les cellules"], ["DeltaV  (mV)", "", "NA", "", "FAIL", "Différence maximale de tension entre les cellules"]] ("Tableau"), "ligne à traiter"=w340) -> ("result string"=w342:string, "Numout"=w336:i32, "errout"=w343:errorcluster)  [unwired: 10 in]
          }
          frame "NULL", Default {
            # "NULL"
          }
        }
      }
    }
  }
  n116 = local read "BDD"() -> (w4:T1)
  n117 = call "DEMO.vi"("errin"=w2, "DATA IN"=w4) -> ("error out"=w1:errorcluster)  [unwired: 9 in]
  n118 = Search and Replace String(replace all?=TRUE ("tout remplacer ? (F)"), input string=w72, search string="<td class=\"core1 testpass\">FAIL</td>" ("chaîne recherchée"), replace string="<td class=\"core1 testfail\">FAIL</td>" ("chaîne de remplacement (\"\")"), error in=w1) -> (result string=w57:string, number of replacements=w52:i32, error out=w68:errorcluster)  [unwired: 3 in, 1 out]
  n119 = Search and Replace String(replace all?=TRUE ("tout remplacer ? (F)"), input string=w57, search string="<td class=\"core1 testpass\">PASS</td>" ("chaîne recherchée"), error in=w68) -> (number of replacements=w60:i32, error out=w64:errorcluster)  [unwired: 4 in, 2 out]
  "nombre de remplacements" <- w60
  n120 = Number To Decimal String(number=w60) -> (decimal integer string=w59:string)  [unwired: 1 in]
  n121 = Number To Decimal String(number=w52) -> (decimal integer string=w58:string)  [unwired: 1 in]
  n122 = Search and Replace String(input string=w57, search string="<!--NBTESTOK-->" ("chaîne recherchée"), replace string=w59, error in=w64) -> (result string=w65:string, error out=w63:errorcluster)  [unwired: 4 in, 2 out]
  n123 = Equal To 0?(x=w52) -> (x = 0?=w44:bool)
  n124 = Search and Replace String(input string=w65, search string="<!--NBTESTKO-->" ("chaîne recherchée"), replace string=w58, error in=w63) -> (result string=w47:string, error out=w51:errorcluster)  [unwired: 4 in, 2 out]
  n125 = Search and Replace String(input string=w47, search string="Résultat du test :\t</td><td class=\"resume5\" colspan=\"3\"><div><span style=\"float:left\" id=\"result\"><font size = \"5pt\" color=\"green\"><b>CONFORME</b>", replace string="Résultat du test :\t</td><td class=\"resume5\" colspan=\"3\"><div><span style=\"float:left\" id=\"result\"><font  size = \"5pt\" color=\"red\"><b>NON CONFORME</b>", error in=w51) -> (result string=w16:string, error out=w50:errorcluster)  [unwired: 4 in, 2 out]
  n126 = Search and Replace String(input string=w16, search string=".resume1,.resume3,.resume4,.resume5,.resume6,.resume7{background-color:#e6feef;padding:7px;border:1px solid black;}\n.resume0{border:1px solid black;background-color:#e6feef;font-weight: bold;padding:0px;text-align: center;}", replace string=".resume1,.resume3,.resume4,.resume5,.resume6,.resume7{background-color:#fdebd0;padding:7px;border:1px solid black;}\n.resume0{border:1px solid black;background-color:#fdebd0;font-weight: bold;padding:0px;text-align: center;}") -> (result string=w15:string)  [unwired: 5 in, 3 out]
  n127 = Select(t=w47, s=w44, f=w15) -> (s? t:f=w48:string)
  "Chaîne" <- w48
  n128 = Not Equal?(x=w6, y=path "") -> (x != y?=w41:bool)
  n129 = Open/Create/Replace File(file path (use dialog)=w73, error in=w50, operation (0:open)=w56) -> (refnum out=w79:refnum<file>, error out=w81:errorcluster)  [unwired: 3 in, 1 out]
  n130 = case shown="True" w41 {
    tunnel: w56 -> [_ w354]
    tunnel: w6 -> [_ w353]
    tunnel: w50 -> [_ w352]
    tunnel: w48 -> [_ w351]
    tunnel: [errorcluster {"status"=FALSE, "code"=0, "source"=""} ("error out") w350] -> w46
    frame False {
    }
    frame True {
      n131 = Open/Create/Replace File(file path (use dialog)=w353, error in=w352, operation (0:open)=w354) -> (refnum out=w355:refnum<file>, error out=w357:errorcluster)  [unwired: 3 in, 1 out]
      n132 = Write to Text File(file (use dialog)=w355, text=w351, error in=w357) -> (refnum out=w356:refnum<file>, error out=w358:errorcluster)  [unwired: 1 in, 1 out]
      n133 = Close File(refnum=w356, error in=w358) -> (error out=w350:errorcluster)  [unwired: 1 out]
    }
  }
  n134 = Write to Text File(file (use dialog)=w79, text=w48, error in=w81) -> (refnum out=w80:refnum<file>, error out=w82:errorcluster)  [unwired: 1 in, 1 out]
  n135 = Close File(refnum=w80, error in=w82) -> (error out=w45:errorcluster)  [unwired: 1 out]
  n136 = Merge Errors(w45, w46) -> (w43:errorcluster)
  "sortie d'erreur" <- w43
  n137 = Compound Arithmetic op=AND ("Opérateur arithmétique")(w44, invert w43) -> (→"tout bon":bool)
